vi "FGV.vi"(8 "error in (no error)":errorcluster, 9 "Actor's Queue In":refnum<class "Message Enqueuer.lvclass">, 10 "Actor name":string, 11 "Action":T2(ring)) -> (0 "error out":errorcluster, 1 "Actor's Queue Out":refnum<class "Message Enqueuer.lvclass">, 2 "Actor names":string[](array[string]))   [LabVIEW 2020, in "Library Commun.lvlib"]
uses:
  <vilib>/ActorFramework/Message Enqueuer/Message Enqueuer.lvclass
  FGV_local.ctl
  Commun VI/TypeDef/Liste Error.ctl
  Commun VI/Library Commun.lvlib
panel:
  in  "FGV_Local":T1
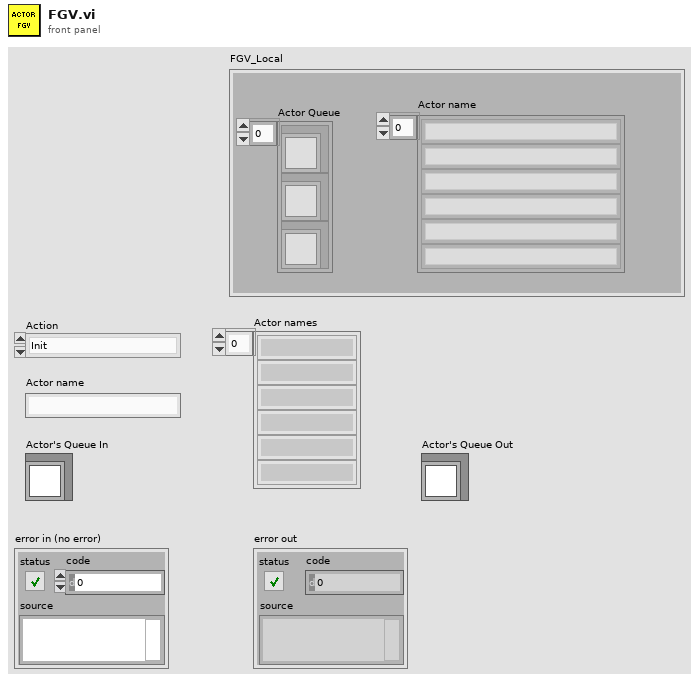
[diagram p1: front panel]
types:
  T1 = typedef "FGV_local.ctl" = cluster{"Actor Queue":refnum<class "Message Enqueuer.lvclass">[], "Actor name":string[]}
  T2 = enum16{"Init", "Add Actor", "Delete Actor", "Get Actor Queue", "Get Log Actor Queue", "List all actors"}
  T3 = typedef "Library Commun.lvlib/Liste Error.ctl" = enum16{"Firebase Driver - Get Document", "Firebase Driver - Get Document With Where", "Firebase Driver - Delete Document", "Firebase Driver - Set Document", "Firebase Driver - Update Document", "Firebase Altyor - Search Document Bench", "Firebase Altyor - Class Not in Firebase", "Spectrum_Analyser - Timeout", "Relay Board - Qty Relay", "DIO - Pb Funtion", "Power_Supply - Peripherical not find", "Mutimeter - Peripherical not find", "Instrument - Function Not Used", "Instrument - Instrument name not specified", "Instrument - Allready Initialised", "Instrument - TimeOut", "Instrument - the instrument must be Initialise before", "Instrument - Frame Not received", "Instrument - Frame Nok", "Test - Initialise the File_for_Save", "Test - Timeout", "Test - Cmd Error", "FGV - Variable ", "BDD FireBase - Define Class", "SN - Class Not Define"}
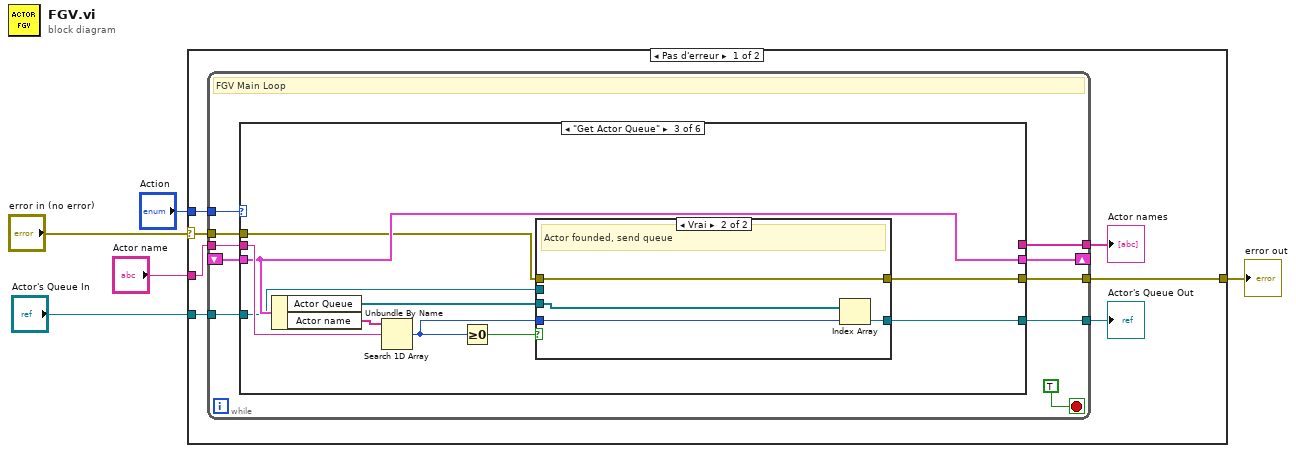
[diagram p0: block diagram]
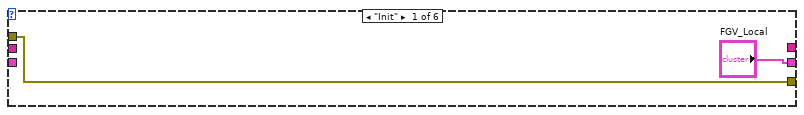
[diagram p2: hidden frame]
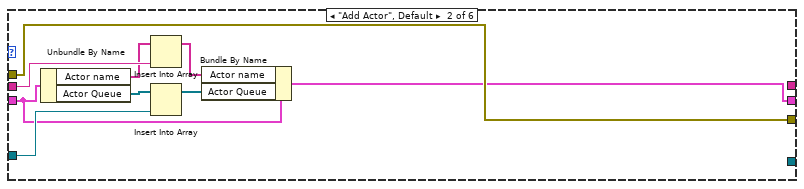
[diagram p3: hidden frame]
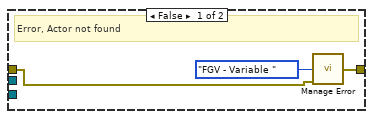
[diagram p4: hidden frame]
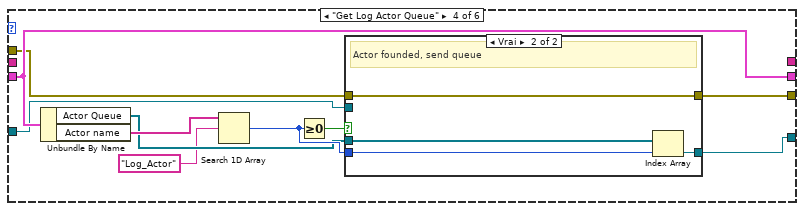
[diagram p5: hidden frame]
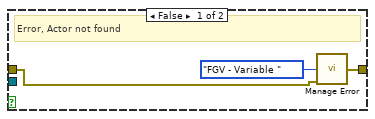
[diagram p6: hidden frame]
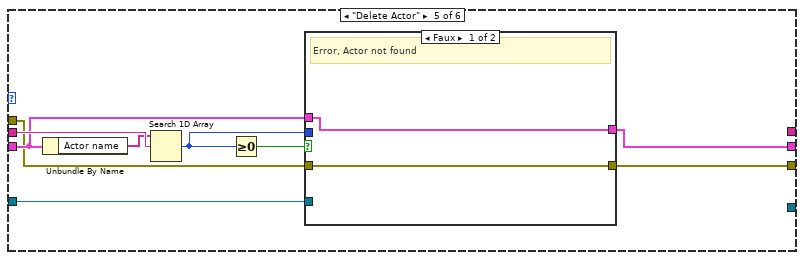
[diagram p7: hidden frame]
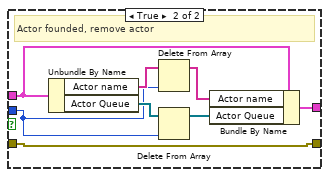
[diagram p8: hidden frame]
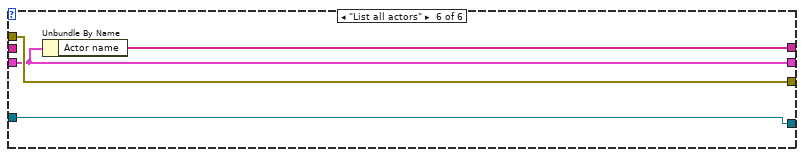
[diagram p9: hidden frame]
diagram:
  n1 = case shown="Pas d'erreur" "error in (no error)" {
    selector: "error in (no error)" -> [w11 w91]
    tunnel: [w10 w91] -> w4
    tunnel: "Action" -> [w12 _]
    tunnel: "Actor name" -> [w9 _]
    tunnel: "Actor's Queue In" -> [w8 _]
    frame No Error {
      n2 = while {
        tunnel: w12 -> [w22]
        tunnel: w11 -> [w21]
        tunnel: [w20] -> w10
        tunnel: w9 -> [w19]
        tunnel: w8 -> [w18]
        shift-right: [w16] -> _
        shift-left: _ -> [w17]
        tunnel: [w15] -> w7
        tunnel: [w13] -> w6
        stop <- TRUE stop-if-true
        # "FGV Main Loop"
        n3 = case shown="\"Get Actor Queue\"" w22 {
          tunnel: w21 -> [w23 w26 w35 w52 w70 w90]
          tunnel: [w23 w26 w34 w51 w68 w90] -> w20
          tunnel: w19 -> [_ w31 w43 _ w76 _]
          tunnel: w18 -> [_ w32 w39 w57 w73 w89]
          tunnel: w17 -> [_ w29 w41 w59 w71 w88]
          tunnel: ["FGV_Local" w25 w41 w59 w69 w88] -> w16
          tunnel: [_ _ w36 w54 _ w89] -> w15
          tunnel: [_ _ _ _ _ w87] -> w13
          frame "Init" {
          }
          frame "Add Actor", Default {
            n4 = Unbundle By Name(w29) -> ("Actor name"=w30:string[], "Actor Queue"=w33:refnum<class "Message Enqueuer.lvclass">[])
            n5 = Insert Into Array(array=w30, new element=w31) -> (w28:string[])  [unwired: 1 in]
            n6 = Insert Into Array(array=w33, new element=w32) -> (w27:refnum<class "Message Enqueuer.lvclass">[])  [unwired: 1 in]
            n7 = Bundle By Name(cluster=w29, "Actor name"=w28, "Actor Queue"=w27) -> (w25:T1)
          }
          frame "Get Actor Queue" {
            n8 = Unbundle By Name(w41) -> ("Actor Queue"=w37:refnum<class "Message Enqueuer.lvclass">[], "Actor name"=w42:string[])
            n9 = Search 1D Array(1D array=w42, element=w43) -> (index of element=w38:i32)  [unwired: 1 in]
            n10 = Greater Or Equal To 0?(x=w38) -> (x >= 0?=w40:bool)
            n11 = case shown="Vrai" w40 {
              tunnel: w39 -> [_ _]
              tunnel: w38 -> [_ w49]
              tunnel: w37 -> [_ w50]
              tunnel: [_ w48] -> w36
              tunnel: w35 -> [w45 w47]
              tunnel: [w44 w47] -> w34
              frame False {
                # "Error, Actor not found"
                n12 = call "Manage Error.vi"("Code Erreur"=Liste_Error."FGV - Variable ", "error in (no error)"=w45) -> ("error out"=w44:errorcluster)  [unwired: 13 in]
              }
              frame True {
                # "Actor founded, send queue"
                n13 = Index Array(array=w50, index=w49) -> (element=w48:refnum<class "Message Enqueuer.lvclass">)
              }
            }
          }
          frame "Get Log Actor Queue" {
            n14 = Unbundle By Name(w59) -> ("Actor Queue"=w55:refnum<class "Message Enqueuer.lvclass">[], "Actor name"=w60:string[])
            n15 = Search 1D Array(1D array=w60, element="Log_Actor") -> (index of element=w56:i32)  [unwired: 1 in]
            n16 = Greater Or Equal To 0?(x=w56) -> (x >= 0?=w58:bool)
            n17 = case shown="Vrai" w58 {
              tunnel: w57 -> [_ _]
              tunnel: w56 -> [_ w66]
              tunnel: w55 -> [_ w67]
              tunnel: [_ w65] -> w54
              tunnel: w52 -> [w62 w64]
              tunnel: [w61 w64] -> w51
              frame False {
                # "Error, Actor not found"
                n18 = call "Manage Error.vi"("Code Erreur"=Liste_Error."FGV - Variable ", "error in (no error)"=w62) -> ("error out"=w61:errorcluster)  [unwired: 13 in]
              }
              frame True {
                # "Actor founded, send queue"
                n19 = Index Array(array=w67, index=w66) -> (element=w65:refnum<class "Message Enqueuer.lvclass">)
              }
            }
          }
          frame "Delete Actor" {
            n20 = Unbundle By Name(w71) -> ("Actor name"=w75:string[])
            n21 = Search 1D Array(1D array=w75, element=w76) -> (index of element=w72:i32)  [unwired: 1 in]
            n22 = Greater Or Equal To 0?(x=w72) -> (x >= 0?=w74:bool)
            n23 = case shown="Faux" w74 {
              tunnel: w73 -> [_ _]
              tunnel: w72 -> [_ w84]
              tunnel: w71 -> [w78 w83]
              tunnel: w70 -> [w77 w79]
              tunnel: [w78 w80] -> w69
              tunnel: [w77 w79] -> w68
              frame False {
                # "Error, Actor not found"
              }
              frame True {
                # "Actor founded, remove actor"
                n24 = Unbundle By Name(w83) -> ("Actor name"=w86:string[], "Actor Queue"=w85:refnum<class "Message Enqueuer.lvclass">[])
                n25 = Delete From Array(array=w86, index=w84) -> (array with subset deleted=w82:string[])  [unwired: 1 in, 1 out]
                n26 = Delete From Array(array=w85, index=w84) -> (array with subset deleted=w81:refnum<class "Message Enqueuer.lvclass">[])  [unwired: 1 in, 1 out]
                n27 = Bundle By Name(cluster=w83, "Actor name"=w82, "Actor Queue"=w81) -> (w80:T1)
              }
            }
          }
          frame "List all actors" {
            n28 = Unbundle By Name(w88) -> ("Actor name"=w87:string[])
          }
        }
      }
      "Actor's Queue Out" <- w7
      "Actor names" <- w6
    }
    frame Error {
    }
  }
  "error out" <- w4
